vi "Text_Create.vi"(0 "reference in":refnum<class "Text.lvclass">, 1 "Object Attributes":T2, 2 "Text Attributes":T1, 5 "error in (no error)":errorcluster) -> (14 "reference out":refnum<class "Text.lvclass">, 19 "error out":errorcluster)   [LabVIEW 2014, in "Text.lvclass"]
uses:
  Text.lvclass
  Object_class/Attributes.ctl
  Object_class/Coordinates.ctl
  Attributes.ctl
  Object_class/Object.lvclass
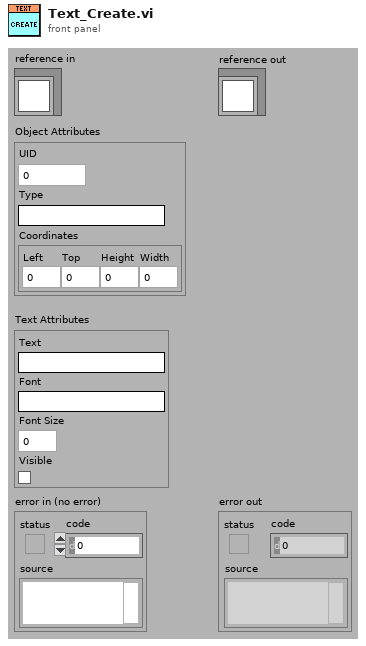
[diagram p1: front panel]
types:
  T1 = typedef "Text.lvclass/Attributes.ctl" = cluster{"Text":string, "Font":string, "Font Size":u32, "Visible":bool}
  T2 = typedef "Object.lvclass/Attributes.ctl" = cluster{"UID":i32, "Type":string, "Coordinates":T3}
  T3 = typedef "Object.lvclass/Coordinates.ctl" = cluster{"Left":i32, "Top":i32, "Height":u32, "Width":u32}
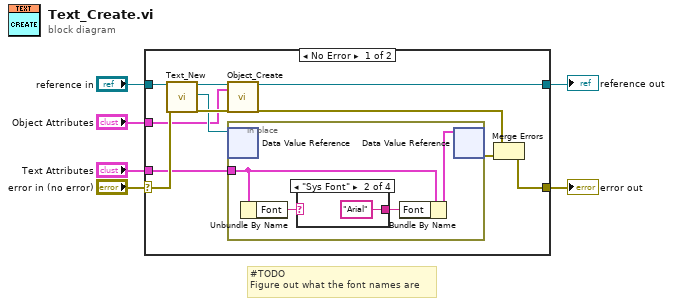
[diagram p0: block diagram]
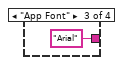
[diagram p3: hidden frame]
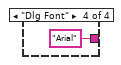
[diagram p4: hidden frame]
diagram:
  # "#TODO\nFigure out what the font names are"
  n1 = case shown="No Error" "error in (no error)" {
    selector: "error in (no error)" -> [w16 w27]
    tunnel: [w14 w27] -> w5
    tunnel: "reference in" -> [w17 w26]
    tunnel: [w11 w26] -> w3
    tunnel: "Object Attributes" -> [w9 _]
    tunnel: "Text Attributes" -> [w8 _]
    frame No Error {
      n2 = call "Text_New.vi"("reference in"=w17, "error in (no error)"=w16) -> ("reference out"=w13:refnum<class "Text.lvclass">, "DVRRefOut"=w10:refnum<data-value>, "error out"=w12:errorcluster)  [unwired: 14 in, 1 out]
      n3 = call "Object_Create.vi"("reference in"=w13, "Object Attributes"=w9, "error in (no error)"=w12) -> ("reference out"=w11:refnum<class "Text.lvclass">, "error out"=w7:errorcluster)  [unwired: 15 in]
      n4 = in-place {
        in-place-border: w8 -> [w20]
        n5 = in-place-dvr #1(w10) -> ()  [unwired: 2 out]
        n6 = Unbundle By Name(w20) -> ("Font"=w21:string)
        n7 = case shown="\"Sys Font\"" w21 {
          selector: w21 -> [w22 _ _ _]
          tunnel: [w22 "Arial" "Arial" "Arial"] -> w18
          frame Default {
          }
          frame "Sys Font" {
          }
          frame "App Font" {
          }
          frame "Dlg Font" {
          }
        }
        n8 = Bundle By Name(cluster=w20, "Font"=w18) -> (w19:T1)
        n9 = in-place-dvr #1(w19) -> (w15:errorcluster)  [unwired: 1 out]
      }
      n10 = Merge Errors(w7, w15) -> (w14:errorcluster)
    }
    frame Error {
    }
  }
  "error out" <- w5
  "reference out" <- w3
